vi "th_update.vi"(2 "th_min":T1, 3 "th_max":T1, 4 "error in (no error)":errorcluster, 5 "th_d":T1, 6 "th[k]":T1, 7 "dt":dbl) -> (0 "error out":errorcluster, 1 "th[k+1]":T1)   [LabVIEW 2021]
uses:
  <vilib>/Analysis/Matrix/Datatypes/RealMatrix.ctl
  <vilib>/Analysis/Matrix/Numeric/Multiply/Multiply - RM,R.vi
  <vilib>/Analysis/Matrix/Numeric/Add/Add - RM,RM.vi
  <vilib>/Analysis/Matrix/NI_Matrix.lvlib
panel:
  out "In Range?":bool[][](array[boolean])
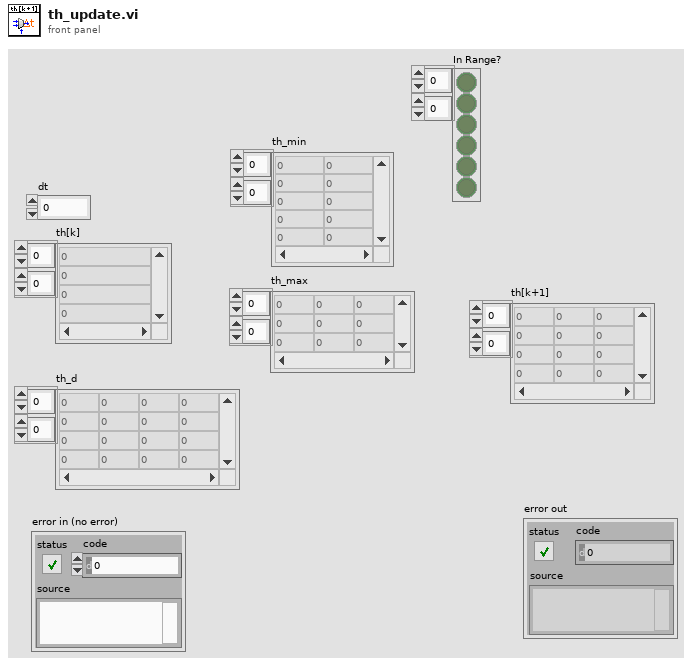
[diagram p1: front panel]
types:
  T1 = typedef "NI_Matrix.lvlib/RealMatrix.ctl" = dbl[][]
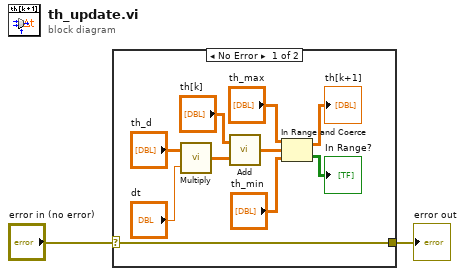
[diagram p0: block diagram]
diagram:
  n1 = case shown="No Error" "error in (no error)" {
    selector: "error in (no error)" -> [w8 w13]
    tunnel: [w8 w13] -> w1
    frame No Error {
      n2 = call-poly <vilib>:"Multiply.vi"("Real Scalar c"="dt", "Real Matrix A"="th_d") -> ("A * c"=w10:T1)
      n3 = call-poly <vilib>:"Add.vi"("Real Matrix B"=w10, "Real Matrix A"="th[k]") -> ("A + B"=w4:T1)
      n4 = In Range and Coerce(upper limit="th_max", x=w4, lower limit="th_min") -> (coerced(x)=→"th[k+1]":dbl[][], In Range?=→"In Range?":bool[][])
    }
    frame Error {
    }
  }
  "error out" <- w1
